vi "Write_StandardInput.vi"(8 "error in (no error)":errorcluster caption="entrée d'erreur (pas d'erreur)", 11 "Process (Default) en entrée":refnum<class "Process (Default).lvclass">) -> (0 "error out":errorcluster caption="sortie d'erreur", 3 "Process (Default) en sortie":refnum<class "Process (Default).lvclass">)   [LabVIEW 2020, in "Library Instrument & Equipement.lvlib" / "Process (Default).lvclass"]
uses:
  Process (Default).lvclass
  Process (Default).lvclass/Process (Default).ctl
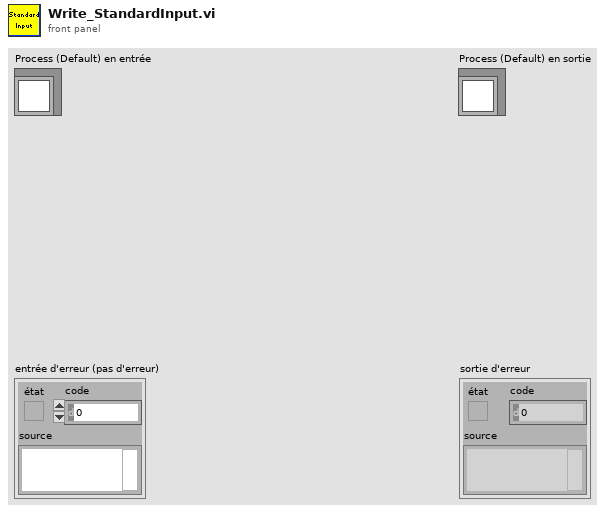
[diagram p1: front panel]
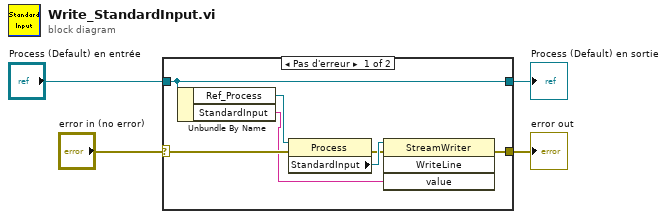
[diagram p0: block diagram]
diagram:
  n1 = case shown="Pas d'erreur" "error in (no error)" {
    selector: "error in (no error)" -> [w7 w13]
    tunnel: [w6 w13] -> w3
    tunnel: [w11 w12] -> w1
    tunnel: "Process (Default) en entrée" -> [w11 w12]
    frame No Error {
      n2 = Unbundle By Name(w11) -> ("Ref_Process"=w10:refnum<k24>, "StandardInput"=w5:string)
      n3 = property on="Nœud de propriété" class="Process"(reference=w10, error in=w7) -> (error out=w8:errorcluster, "StandardInput"=w9:refnum<k24>)  [unwired: 1 out]
      n4 = invoke class="StreamWriter" method="WriteLine"(reference=w9, error in=w8, "value"=w5) -> (error out=w6:errorcluster)  [unwired: 1 in, 3 out]
    }
    frame Error {
    }
  }
  "error out" <- w3
  "Process (Default) en sortie" <- w1
